vi "ReverseData.vi"(1 "Array in":i16[][](array[numeric])) -> (0 "Array out":i16[][](array[numeric]))   [LabVIEW 2022 SP3]
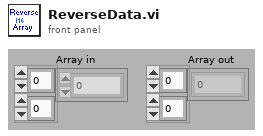
[diagram p1: front panel]
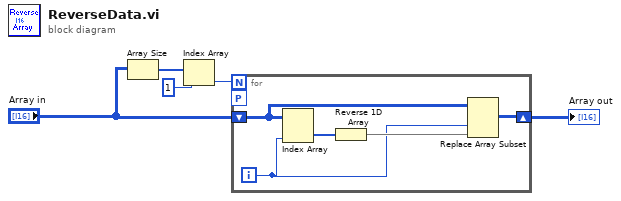
[diagram p0: block diagram]
diagram:
  n1 = Array Size(array="Array in") -> (size(s)=w3:i32[])
  n2 = Index Array(array=w3, index=1) -> (element=w1:i32)
  n3 = for {
    N: w1 -> [_]
    shift-right: [w9] -> w5
    shift-left: "Array in" -> [w8]
    workers-P: _ -> [_]
    i -> [w6]
    n4 = Index Array(array=w8, index (col)=w6) -> (element=w10:i16[])  [unwired: 1 in]
    n5 = Reverse 1D Array(array=w10) -> (reversed array=w7:i16[])
    n6 = Replace Array Subset(array=w8, new element=w7, index (col)=w6) -> (w9:i16[][])  [unwired: 1 in]
  }
  "Array out" <- w5
